vi "EOL_TDKData.vi"(8 "Exit Program":refnum<vi>, 9 "Voltage":dbl=13.5, 10 "idx":u16, 11 "VISA name":refnum<visa-resource-name>) -> ()   [LabVIEW 2018]
uses:
  Def Ctrl/TestSeq.ctl
  <vilib>/Instr/_visa.llb/VISA Configure Serial Port (Instr).vi
  Data buffer/ST0 current buffer.vi
  Data buffer/ST1 current buffer.vi
  Data buffer/ST2 current buffer.vi
  Data buffer/ST3 current buffer.vi
  Data buffer/ST4 current buffer.vi
  Data buffer/ST5 current buffer.vi
panel:
  out "Max Cur":dbl
  out "Cur":dbl
  in  "General Settings:Timeout Value":u32=2000
  in  "flow control (0:none)":u16(ring)=1 caption="流控制（0:无）" items=["无", "XON/XOFF", "RTS/CTS", "XON/XOFF & RTS/CTS", "DTR/DSR", "XON/XOFF & DTR/DSR"]
  out "loss?":bool
  out "Packet loss":i32
  out "current":dbl(graph)
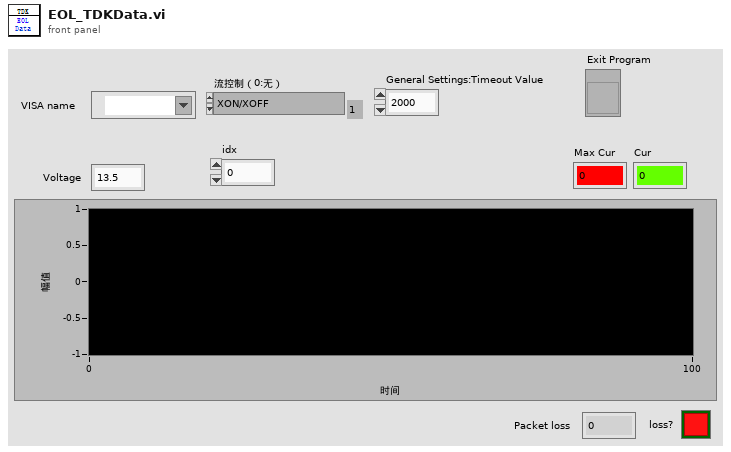
[diagram p1: front panel]
types:
  T1 = typedef "TestSeq.ctl" = enum16{"Idle", "Re Connect", "Error", "Initial", "Set Voltage", "Set Current", "Set Out", "Check Voltage", "Check Current", "Check Version No", "Check Out", "Get Current Data", "EOL Get Current Data"}
  T2 = cluster{"VISA name":refnum<visa-resource-name>, "MsgRec":string, "Current buffer":dbl[], "Timer":i32, "CycleNumb":i32, "Error":errorcluster, "Max Cur":dbl}
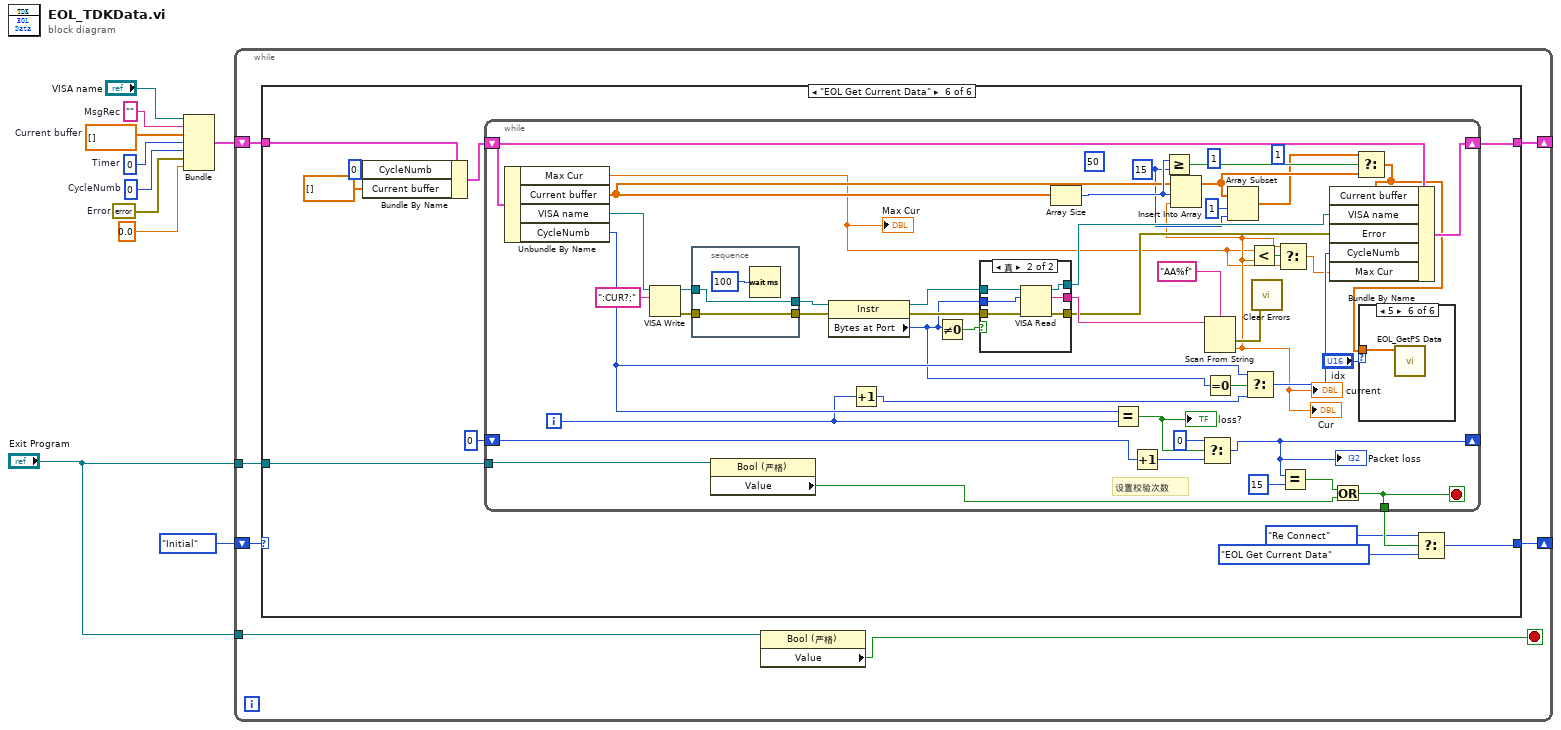
[diagram p0: block diagram]
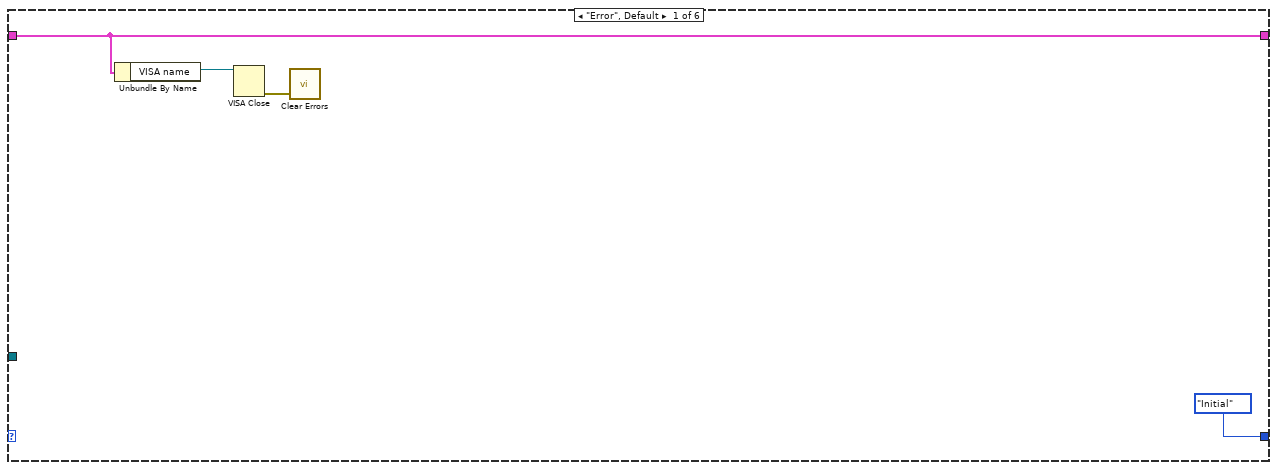
[diagram p2: hidden frame]
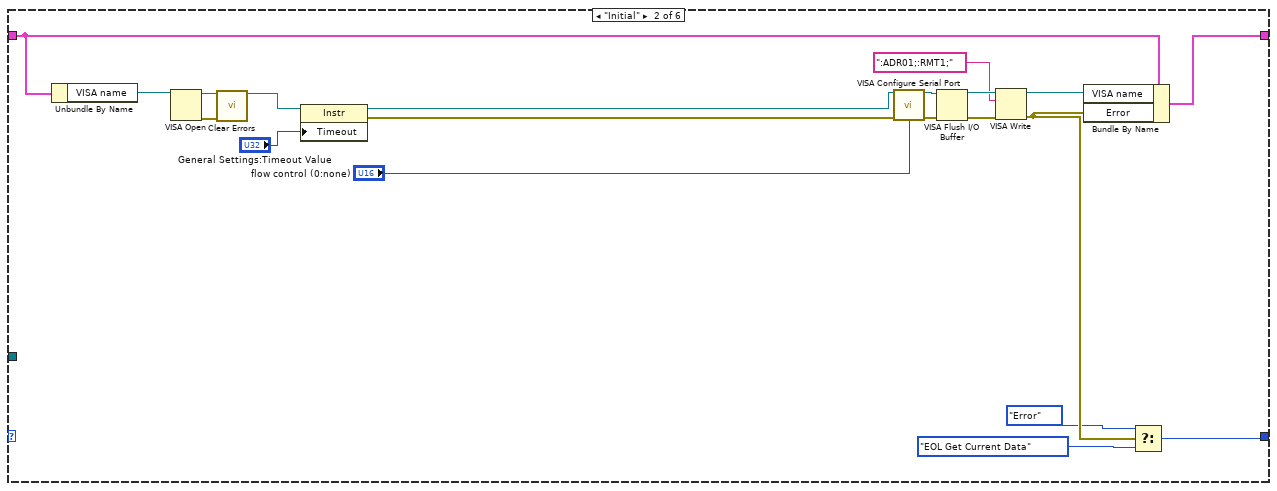
[diagram p3: hidden frame]
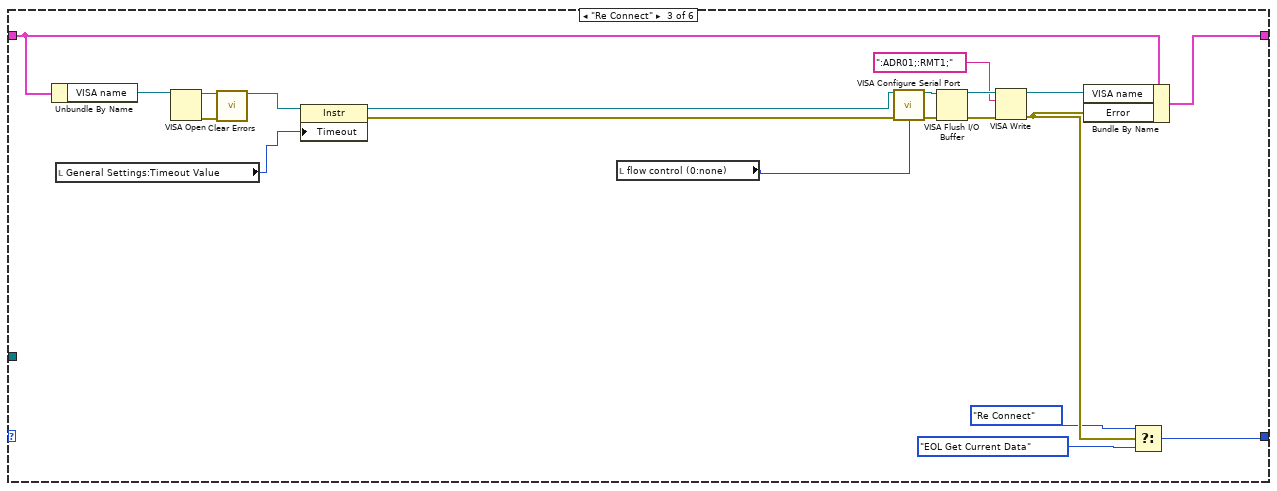
[diagram p4: hidden frame]
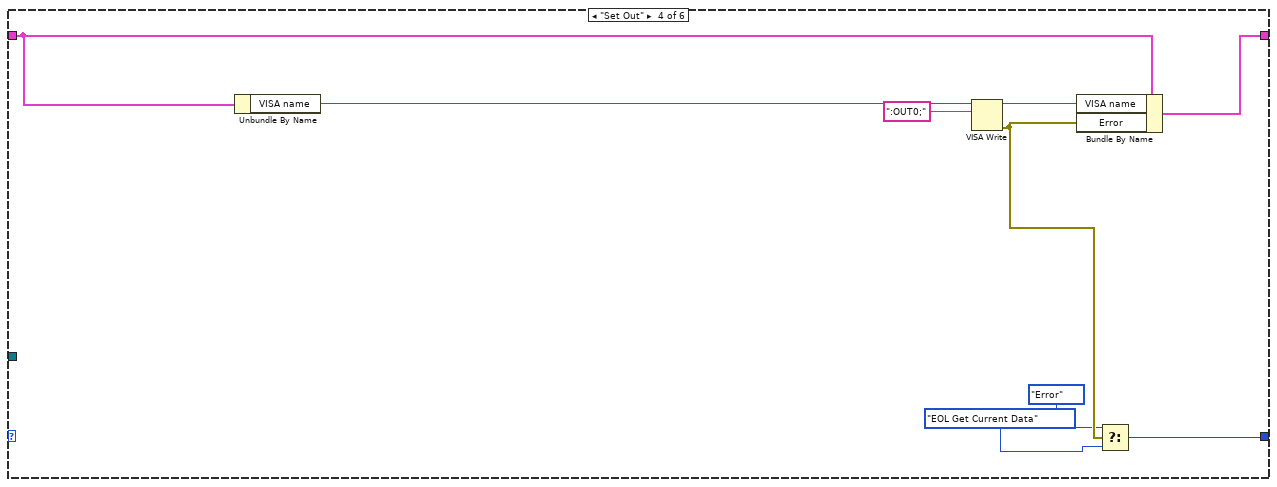
[diagram p5: hidden frame]
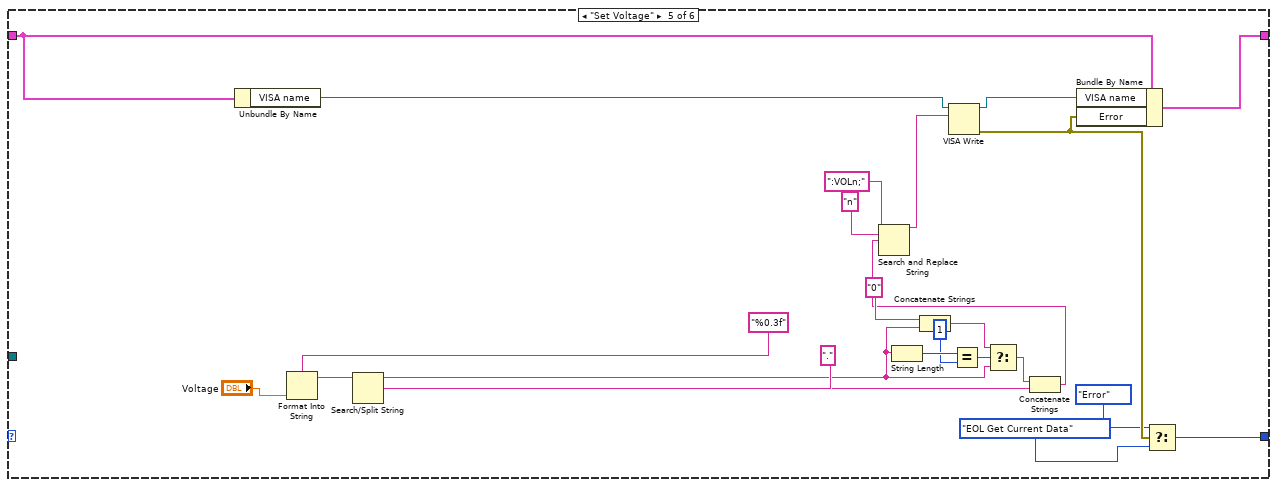
[diagram p6: hidden frame]
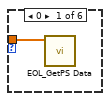
[diagram p7: hidden frame]
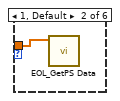
[diagram p8: hidden frame]
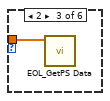
[diagram p9: hidden frame]
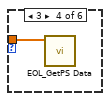
[diagram p10: hidden frame]
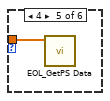
[diagram p11: hidden frame]
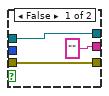
[diagram p12: hidden frame]
diagram:
  w3 = errorcluster {"status"=FALSE, "code"=0, "source"=""}  # Error
  w6 = 0  # CycleNumb
  w7 = 0  # Timer
  w10 = ""  # MsgRec
  w9 = dbl[] []  # Current buffer
  n1 = Bundle("VISA name"="VISA name", "MsgRec"=w10, "Current buffer"=w9, "Timer"=w7, "CycleNumb"=w6, "Error"=w3, "Max Cur"=0.0) -> (w5:T2)  [unwired: 1 in]
  n2 = while {
    shift-right: [w15] -> _
    shift-left: w5 -> [w16]
    shift-right: [w14] -> _
    shift-left: TestSeq."Initial" -> [w17]
    tunnel: "Exit Program" -> [w12]
    tunnel: "Exit Program" -> [w11]
    stop <- w13 stop-if-true
    n3 = case shown="\"EOL Get Current Data\"" w17 {
      tunnel: w16 -> [w19 w40 w59 w68 w92 w99]
      tunnel: [w19 w39 w58 w67 w91 w102] -> w15
      tunnel: [TestSeq."Initial" w24 w45 w61 w70 w95] -> w14
      tunnel: w11 -> [_ _ _ _ _ w93]
      frame "Error", Default {
        n4 = Unbundle By Name(w19) -> ("VISA name"=w20:refnum<visa-resource-name>)
        n5 = VISA Close(VISA resource name=w20) -> (error out=w18:errorcluster)  [unwired: 1 in]
        n6 = call <vilib>:"Clear Errors.vi"("error in (no error)"=w18) -> ()  [unwired: 5 in, 2 out]
      }
      frame "Initial" {
        n7 = Unbundle By Name(w40) -> ("VISA name"=w31:refnum<visa-resource-name>)
        n8 = VISA Open(VISA resource name=w31) -> (VISA resource name=w36:refnum<visa-resource-name>, error out=w22:errorcluster)  [unwired: 4 in]
        n9 = call <vilib>:"Clear Errors.vi"("error in (no error)"=w22) -> ()  [unwired: 5 in, 2 out]
        n10 = property class="Instr"(reference=w36, "Timeout"="General Settings:Timeout Value") -> (reference out=w35:refnum<visa-resource-name>, error out=w34:errorcluster)  [unwired: 1 in]
        n11 = call-poly "VISA Configure Serial Port"("VISA resource name"=w35, "error in (no error)"=w34, "flow control (0:none)"="flow control (0:none)") -> ("VISA resource name out"=w37:refnum<visa-resource-name>, "error out"=w38:errorcluster)  [unwired: 11 in]
        n12 = VISA Flush I/O Buffer(VISA resource name=w37, error in (no error)=w38) -> (VISA resource name out=w30:refnum<visa-resource-name>, error out=w29:errorcluster)  [unwired: 1 in]
        n13 = VISA Write(VISA resource name=w30, write buffer=":ADR01;:RMT1;" ("Command Out"), error in (no error)=w29) -> (VISA resource name out=w27:refnum<visa-resource-name>, error out=w26:errorcluster)  [unwired: 1 out]
        n14 = Bundle By Name(cluster=w40, "VISA name"=w27, "Error"=w26) -> (w39:T2)
        n15 = Select(t=TestSeq."Error", s=w26, f=TestSeq."EOL Get Current Data") -> (s? t:f=w24:T1)
      }
      frame "Re Connect" {
        n16 = Unbundle By Name(w59) -> ("VISA name"=w52:refnum<visa-resource-name>)
        n17 = local read "General Settings:Timeout Value"() -> (w41:u32)
        n18 = VISA Open(VISA resource name=w52) -> (VISA resource name=w55:refnum<visa-resource-name>, error out=w43:errorcluster)  [unwired: 4 in]
        n19 = call <vilib>:"Clear Errors.vi"("error in (no error)"=w43) -> ()  [unwired: 5 in, 2 out]
        n20 = property class="Instr"(reference=w55, "Timeout"=w41) -> (reference out=w54:refnum<visa-resource-name>, error out=w53:errorcluster)  [unwired: 1 in]
        n21 = local read "flow control (0:none)"() -> (w42:u16)
        n22 = call-poly "VISA Configure Serial Port"("VISA resource name"=w54, "error in (no error)"=w53, "flow control (0:none)"=w42) -> ("VISA resource name out"=w56:refnum<visa-resource-name>, "error out"=w57:errorcluster)  [unwired: 11 in]
        n23 = VISA Flush I/O Buffer(VISA resource name=w56, error in (no error)=w57) -> (VISA resource name out=w51:refnum<visa-resource-name>, error out=w50:errorcluster)  [unwired: 1 in]
        n24 = VISA Write(VISA resource name=w51, write buffer=":ADR01;:RMT1;" ("Command Out"), error in (no error)=w50) -> (VISA resource name out=w48:refnum<visa-resource-name>, error out=w47:errorcluster)  [unwired: 1 out]
        n25 = Bundle By Name(cluster=w59, "VISA name"=w48, "Error"=w47) -> (w58:T2)
        n26 = Select(t=TestSeq."Re Connect", s=w47, f=TestSeq."EOL Get Current Data") -> (s? t:f=w45:T1)
      }
      frame "Set Out" {
        n27 = Unbundle By Name(w68) -> ("VISA name"=w66:refnum<visa-resource-name>)
        n28 = VISA Write(VISA resource name=w66, write buffer=":OUT0;" ("写入缓冲区")) -> (VISA resource name out=w64:refnum<visa-resource-name>, error out=w63:errorcluster)  [unwired: 1 in, 1 out]
        n29 = Bundle By Name(cluster=w68, "VISA name"=w64, "Error"=w63) -> (w67:T2)
        n30 = Select(t=TestSeq."Error", s=w63, f=TestSeq."EOL Get Current Data") -> (s? t:f=w61:T1)
      }
      frame "Set Voltage" {
        n31 = Unbundle By Name(w92) -> ("VISA name"=w75:refnum<visa-resource-name>)
        n32 = Format Into String(format string="%0.3f" ("Command Out"), "Voltage") -> (resulting string=w88:string)  [unwired: 2 in, 1 out]
        n33 = Search/Split String(string=w88, search string/char (-)=".") -> (substring before match=w82:string, match + rest of string=w80:string)  [unwired: 1 in, 1 out]
        n34 = String Length(string=w82) -> (length=w87:i32)
        n35 = Concatenate Strings("0" ("string"), w82) -> (w84:string)
        n36 = Equal?(x=w87, y=1) -> (x = y?=w85:bool)
        n37 = Select(t=w84, s=w85, f=w82) -> (s? t:f=w81:string)
        n38 = Concatenate Strings(w81, w80) -> (w78:string)
        n39 = Search and Replace String(input string=":VOLn;" ("输入字符串"), search string="n" ("搜索字符串"), replace string=w78) -> (result string=w74:string)  [unwired: 5 in, 3 out]
        n40 = VISA Write(VISA resource name=w75, write buffer=w74) -> (VISA resource name out=w73:refnum<visa-resource-name>, error out=w72:errorcluster)  [unwired: 1 in, 1 out]
        n41 = Bundle By Name(cluster=w92, "VISA name"=w73, "Error"=w72) -> (w91:T2)
        n42 = Select(t=TestSeq."Error", s=w72, f=TestSeq."EOL Get Current Data") -> (s? t:f=w70:T1)
      }
      frame "EOL Get Current Data" {
        n43 = Bundle By Name(cluster=w99, "CycleNumb"=0, "Current buffer"=dbl[] []) -> (w98:T2)
        n44 = while {
          shift-right: [w146] -> w102
          shift-left: w98 -> [w147]
          shift-right: [w136] -> _
          shift-left: 0 -> [w143]
          tunnel: [w109] -> w97
          tunnel: w93 -> [w112]
          i -> [w115]
          stop <- w109 stop-if-true
          (unwired) 50 ("y")
          (unwired) 1 ("长度")
          (unwired) 1 ("索引")
          w118 = 15 ("y")
          # "设置校验次数"
          n45 = Unbundle By Name(w147) -> ("Max Cur"=w105:dbl, "Current buffer"=w137:dbl[], "VISA name"=w126:refnum<visa-resource-name>, "CycleNumb"=w145:i32)
          "Max Cur" <- w105
          n46 = VISA Write(VISA resource name=w126, write buffer=":CUR?;" ("写入缓冲区")) -> (VISA resource name out=w132:refnum<visa-resource-name>, error out=w133:errorcluster)  [unwired: 1 in, 1 out]
          n47 = stacked-sequence {
            tunnel: w132 -> [w165]
            tunnel: [w165] -> w131
            tunnel: w133 -> [w164]
            tunnel: [w164] -> w130
            frame #0 {
              n48 = Wait (ms)(milliseconds to wait=u32 100) -> ()  [unwired: 1 out]
            }
          }
          n49 = property class="Bool (严格)"(reference=w112) -> ("Value"=w110:bool)  [unwired: 1 in, 2 out]
          n50 = property class="Instr"(reference=w131, error in=w130) -> (reference out=w129:refnum<visa-resource-name>, error out=w128:errorcluster, "Bytes at Port"=w124:u32)
          n51 = Increment(x=w115) -> (x+1=w114:i32)
          n52 = Not Equal To 0?(x=w124) -> (x != 0?=w127:bool)
          n53 = case shown="真" w127 {
            tunnel: [w155 w163] -> w123
            tunnel: [w156 w162] -> w122
            tunnel: ["" ("read buffer") w161] -> w125
            tunnel: w129 -> [w156 w160]
            tunnel: w128 -> [w155 w159]
            tunnel: w124 -> [_ w158]
            frame False {
            }
            frame True {
              n54 = VISA Read(VISA resource name=w160, byte count=w158, error in (no error)=w159) -> (VISA resource name out=w162:refnum<visa-resource-name>, read buffer=w161:string, error out=w163:errorcluster)  [unwired: 1 out]
            }
          }
          n55 = Array Size(array=w137) -> (size(s)=w138:i32)
          n56 = Equal?(x=w145, y=w115) -> (x = y?=w135:bool)
          "loss?" <- w135
          n57 = Increment(x=w143) -> (x+1=w144:i32)
          n58 = Greater Or Equal?(x=w138, y=w118) -> (x >= y?=w139:bool)
          n59 = Select(t=0, s=w135, f=w144) -> (s? t:f=w136:i32)
          "Packet loss" <- w136
          n60 = Scan From String(format string="AA%f" ("格式字符串"), input string=w125) -> (error out=w140:errorcluster, output 1=w106:dbl)  [unwired: 3 in, 2 out]
          "current" <- w106
          "Cur" <- w106
          n61 = Insert Into Array(array=w137, index=w138, new element=w106) -> (w116:dbl[])
          n62 = Equal To 0?(x=w124) -> (x = 0?=w148:bool)
          n63 = Array Subset(array=w116, index=1 ("索引"), length=w118) -> (w113:dbl[])
          n64 = Select(t=w145, s=w148, f=w114) -> (s? t:f=w134:i32)
          n65 = Less?(x=w105, y=w106) -> (x < y?=w107:bool)
          n66 = call <vilib>:"Clear Errors.vi"("error in (no error)"=w140) -> ()  [unwired: 5 in, 2 out]
          n67 = Select(t=w106, s=w107, f=w105) -> (s? t:f=w104:dbl)
          n68 = Equal?(x=w136, y=15) -> (x = y?=w111:bool)
          n69 = Or(x=w111, y=w110) -> (x .or. y?=w109:bool)
          n70 = Select(t=w113, s=w139, f=w116) -> (s? t:f=w117:dbl[])
          n71 = Bundle By Name(cluster=w147, "Current buffer"=w117, "VISA name"=w122, "Error"=w123, "CycleNumb"=w134, "Max Cur"=w104) -> (w146:T2)
          n72 = case shown="5" "idx" {
            tunnel: w117 -> [w149 w150 w151 w152 w153 w154]
            frame 0 {
              n73 = call-poly "EOL_GetPS Data.vi"("in"=w149) -> ()  [unwired: 9 in, 2 out]
            }
            frame 1, Default {
              n74 = call-poly "EOL_GetPS Data.vi"("in"=w150) -> ()  [unwired: 9 in, 2 out]
            }
            frame 2 {
              n75 = call-poly "EOL_GetPS Data.vi"("in"=w151) -> ()  [unwired: 9 in, 2 out]
            }
            frame 3 {
              n76 = call-poly "EOL_GetPS Data.vi"("in"=w152) -> ()  [unwired: 9 in, 2 out]
            }
            frame 4 {
              n77 = call-poly "EOL_GetPS Data.vi"("in"=w153) -> ()  [unwired: 9 in, 2 out]
            }
            frame 5 {
              n78 = call-poly "EOL_GetPS Data.vi"("in"=w154) -> ()  [unwired: 9 in, 2 out]
            }
          }
        }
        n79 = Select(t=TestSeq."Re Connect", s=w97, f=TestSeq."EOL Get Current Data") -> (s? t:f=w95:T1)
      }
    }
    n80 = property class="Bool (严格)"(reference=w12) -> ("Value"=w13:bool)  [unwired: 1 in, 2 out]
  }
